vi "MiniBatchSparsePCA.vi"(8 "error in":errorcluster) -> (0 "error out":errorcluster, 3 "out":refnum<class "MiniBatchSparsePCA.lvclass">)   [LabVIEW 2020]
doc: "Mini-batch Sparse Principal Components Analysis\n\n Finds the set of sparse components that can optimally reconstruct\n the data. The amount of sparseness is controllable by the coefficient\n of the L1 penalty, given by the parameter alpha.\n\n Read more in the :ref:`User Guide <SparsePCA>`.\n\n Parameters\n ----------\n n_components : int, default=None\n number of sparse atoms to extract\n\n alpha : int, default=1\n Sparsity controlling parameter. Higher values lead to sparser\n components.\n\n ridge_alpha : float, default=0.01\n Amount of ridge shrinkage to apply in order to improve\n conditioning when calling the transform method.\n\n n_iter : int, default=100\n number of iterations to perform for each mini batch\n\n callback : callable, default=None\n callable that gets invoked every five iterations\n\n batch_size : int, default=3\n the number of features to take in each mini batch\n\n verbose : int or bool, default=False\n Controls the verbosity; the higher, the more messages. Defaults to 0.\n\n shuffle : bool, default=True\n whether to shuffle the data before splitting it in batches\n\n n_jobs : int, default=None\n Number of parallel jobs to run.\n ``None`` means 1 unless in a :obj:`joblib.parallel_backend` context.\n ``-1`` means using all processors. See :term:`Glossary <n_jobs>`\n for more details.\n\n method : {'lars', 'cd'}, default='lars'\n lars: uses the least angle regression method to solve the lasso problem\n (linear_model.lars_path)\n cd: uses the coordinate descent method to compute the\n Lasso solution (linear_model.Lasso). Lars will be faster if\n the estimated components are sparse.\n\n random_state : int, RandomState instance or None, default=None\n Used for random shuffling when ``shuffle`` is set to ``True``,\n during online dictionary learning. Pass an int for reproducible results\n across multiple function calls.\n See :term:`Glossary <random_state>`.\n\n Attributes\n ----------\n components_ : ndarray of shape (n_components, n_features)\n Sparse components extracted from the data.\n\n n_components_ : int\n Estimated number of components.\n\n .. versionadded:: 0.23\n\n n_iter_ : int\n Number of iterations run.\n\n mean_ : ndarray of shape (n_features,)\n Per-feature empirical mean, estimated from the training set.\n Equal to ``X.mean(axis=0)``.\n\n \nAvailable methods:\nFit\nFit Transform\nTransform\nGet Attributes\nGet Params\nSet Params"
uses:
  MiniBatchSparsePCA.lvclass
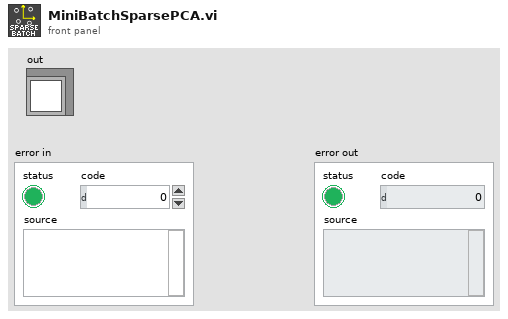
[diagram p1: front panel]
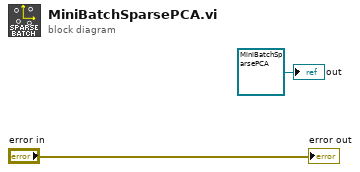
[diagram p0: block diagram]
diagram:
  "out" <- refnum<class "MiniBatchSparsePCA.lvclass"> refnum ("model")
  "error out" <- "error in"
